vi "TEST SCREEN UPDATE.vi"(0 "Staion  in 1":refnum<k5>, 2 "Staion  in 2":refnum<k5>, 3 "Staion  in error 2":errorcluster, 4 "Staion  in 3":refnum<k5>, 5 "Staion  in error 3":errorcluster, 6 "DataBase connection in":T10, 7 "Database error in":errorcluster, 21 "Staion  in error 1":errorcluster) -> (1 "Staion Error Out 1":errorcluster, 20 "Staion Out 1":refnum<k5>, 22 "Staion Out 2":refnum<k5>, 23 "Staion Error Out 2":errorcluster, 24 "Staion Out 3":refnum<k5>, 25 "Staion Error Out 3":errorcluster, 26 "Database connection out":T10, 27 "Database error out":errorcluster)   [LabVIEW 2024]
uses:
  <vilib>/addons/database/Connection.llb/Conn ObjectReference.ctl
  Controls/OP10_Cluster.ctl
  Controls/OP20_Cluster.ctl
  Controls/OP30_Cluster.ctl
  Controls/OP30_1_Cluster.ctl
  Controls/OP40_1_Cluster.ctl
  Controls/OP40_Cluster.ctl
  Controls/OP40_2_Cluster.ctl
  Controls/OP40_3_Cluster.ctl
  Controls/Data_Cluster_1.ctl
  test sequnece leak.ctl
  test setting.ctl
  Data base/database cluster.ctl
  Variable/Global.vi
  Support/Message Queue/Message Queue.lvlib
  <vilib>/addons/database/NI_Database_API.lvlib
panel:
  in  "Exit":bool
  in  "Tab Control":enum32{"Screen_1", "Screen_2", "Other"}(tab)
  out "OP_30_1":T1
  out "OP_30":T2
  out "OP_20":T3
  out "OP_10":T4
  out "Result":string[][](table)
  out "OP_40_3":T5
  out "OP_40_2":T6
  out "OP_40":T7
  out "OP_40_1":T8
  in  "Tab Control 2":enum32{"OP_10", "OP_20", "OP_30", "OP_40"}(tab)
  out "OP_10":string[](array[string])
  in  "Barcode OK":bool
  in  "Barcode NG":bool
  in  "Barcode Already":bool
  in  "M 1":T9
  out "OP_10":u16[][](array[numeric])
  out "OP_10":sgl[][](array[numeric])
  in  "Barcode Already 2":bool
  in  "Barcode NG 2":bool
  in  "Barcode OK 2":bool
  in  "M 2":T9
  out "OP_20":string[](array[string])
  out "OP_20":u16[][](array[numeric])
  out "OP_20":sgl[][](array[numeric])
  in  "M 3":T9
  in  "Barcode Already 3":bool
  in  "Barcode NG 3":bool
  in  "Barcode OK 3":bool
  out "OP_30":string[](array[string])
  out "OP_30":u16[][](array[numeric])
  out "OP_30":sgl[][](array[numeric])
  in  "M 4":T9
  in  "Barcode Already 4":bool
  in  "Barcode NG 4":bool
  in  "Barcode OK 4":bool
  out "OP_40":string[](array[string])
  out "OP_40":sgl[][](array[numeric])
  out "OP_40":u16[][](array[numeric])
  out "sr. out BARCODE":i32
  out "sr. out Laser":i32
  out "length":i32
  out "CommLoopCount":i32
  out "Communication error 3":bool
  out "Communication error 2":bool
  out "Communication error 1":bool
  out "path for Laser sr":path
  out "path for Barcode sr.":path
  in  "Model NAME":string
  in  "count Path":path=path "D:/Configuration Folder Barcode/srno"
  in  "Visible":bool
  out "Exit 3":bool
  in  "TEST SETTING PATH":path=path "D:/Data Actuator/config/Settings"
  in  "Setting":path=path "D:/data/Test Settings"
  # "Test Screen"
  # "TESTING DATALOGGING SYSTEM"
  # "Station  OP 10"
  # "Station  OP 20"
  # "Station  OP 30"
  # "Station  OP 30_1"
  # "Station  OP 40"
  # "Station  OP 40_1"
  # "Station  OP 40_2"
  # "Station  OP 40_3"
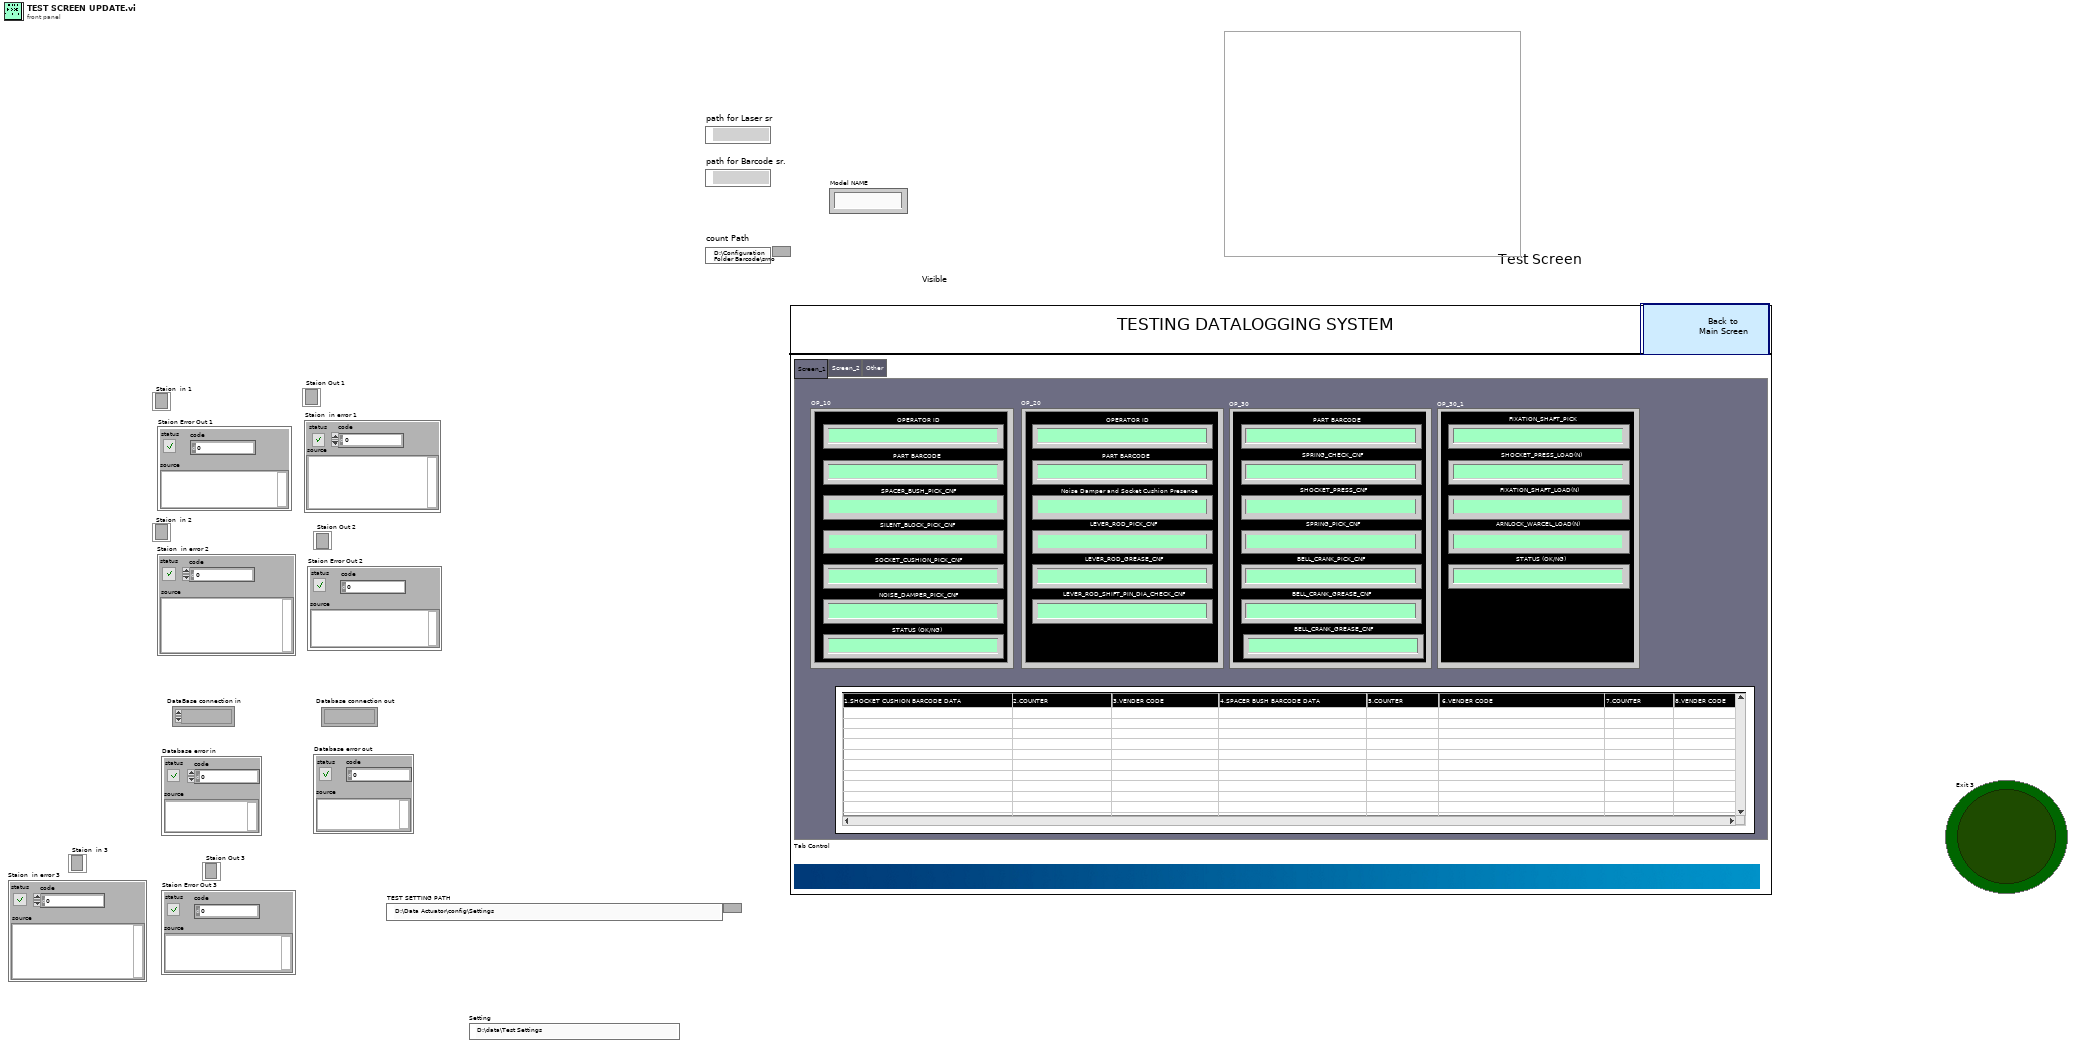
[diagram p1: front panel]
types:
  T1 = typedef "OP30_1_Cluster.ctl" = cluster{"SHOCKET_PRESS_LOAD(N) ":string, "FIXATION_SHAFT_PICK   ":string, "FIXATION_SHAFT_LOAD(N)":string, "ARNLOCK_WARCEL_LOAD(N)":string, "STATUS (OK/NG)":string}
  T2 = typedef "OP30_Cluster.ctl" = cluster{"SPRING_CHECK_CNF ":string, "PART BARCODE  ":string, "SHOCKET_PRESS_CNF":string, "SPRING_PICK_CNF":string, "BELL_CRANK_PICK_CNF":string, "BELL_CRANK_GREASE_CNF":string, "BELL_CRANK_GREASE_CNF":string}
  T3 = typedef "OP20_Cluster.ctl" = cluster{"PART BARCODE ":string, "OPERATOR ID ":string, "Noise Damper and Socket Cushion Presence":string, "LEVER_ROD_PICK_CNF":string, "LEVER_ROD_GREASE_CNF":string, "LEVER_ROD_SHIFT_PIN_DIA_CHECK_CNF":string}
  T4 = typedef "OP10_Cluster.ctl" = cluster{"OPERATOR ID ":string, "PART BARCODE ":string, "SPACER_BUSH_PICK_CNF":string, "SILENT_BLOCK_PICK_CNF":string, "SOCKET_CUSHION_PICK_CNF":string, "NOISE_DAMPER_PICK_CNF":string, "STATUS (OK/NG)":string}
  T5 = typedef "OP40_3_Cluster.ctl" = cluster{"SELECT_5TH_REV_LOAD(N) ":string, "SELECT_1ST_2ND_LOAD(N)":string, "HYSTERISIS CONFIRMATION":string, "PUNCH CONFIRMATION":string, "PDI FIXTURE CONFIRMATION":string, "EOL OK BARCODE SCAN CNF":string, "STATUS (OK/NG)":string}
  T6 = typedef "OP40_2_Cluster.ctl" = cluster{"SHIFT_2ND_4TH_REV_TRAVEL ":string, "PART BARCODE ":string, "SHIFT_1ST_3RD_5TH_TRAVEL ":string, "SHIFT_2ND_4TH_REV_LOAD(N)":string, "SHIFT_1ST_3RD_5TH_LOAD(N)":string, "SELECT_1ST_2ND_TRAVEL":string, "SELECT_5TH_REV_TRAVEL":string}
  T7 = typedef "OP40_Cluster.ctl" = cluster{"PART BARCODE ":string, "OPERATOR ID ":string, "BOOT_ORIENTATION_CHECK_CNF":string, "3_BOND_CONFIRMATION":string, "STATUS (OK/NG)":string, "PRETIGHT ANGLE":string, "POST TIGHT ANGLE":string}
  T8 = typedef "OP40_1_Cluster.ctl" = cluster{"MAX KNOB TORQUE ":string, "KNOB TIGHT BARCODE OK ":string, "NO. OF TURNS":string, "HEIGHT CHECK":string, "2 MM GAUGE CHECK":string, "STATUS (OK/NG)":string, "OPERATOR ID":string}
  T9 = cluster{"Test Start Leak":bool, "Test Stop Leak":bool, "Scan Barcode":bool, "Test Running":bool, "Test OK":bool, "Test NG":bool, "Spare 1":bool, "Spare 2":bool}
  T10 = typedef "NI_Database_API.lvlib/Conn ObjectReference.ctl" = refnum<k1>
  T11 = typedef "Data_Cluster_1.ctl" = cluster{"OP_10":T4}
  T12 = enum16{"open", "replace", "create", "open or create", "replace or create", "replace or create with confirmation"}
  T13 = typedef "test setting.ctl" = cluster{"M&M Part No.":string, "Vendor Code":string, "Part Identification Code":string, "Next Barcode Printing Wait Time":i32, "Path for LAser":path}
  T14 = typedef "test sequnece leak.ctl" = enum16{"Intilize", "CYCLE RESET", "Wait For teststart", "wait for scan", "check Barcode", "wait for start", "Wait for result", "wait for complete", "test stop", "Wait for LAser Scan Data", "check Scan Laser Data", "data save", "update tabel", "send data to Laser", "wait for Laser Start", "wait for laser stop"}
  T15 = typedef "database cluster.ctl" = cluster{"ID":i64, "Datetime":string, "PARTBARCODE":string, "TORQUE":string, "RESULT1":string, "CHILD1":string, "CHILD2":string, "CHILD3":string, "CHILD4":string, "RESULT2":string, "FINALBARCODE":string, "RESULT3":string, "REMARK":string, "OTHER":string}
  T16 = typedef "Communication setting.ctl" = cluster{"Light Scanner Port":refnum<visa-resource-name>, "Shift-A":timestamp, "Shift-B":timestamp, "Shift-C":timestamp, "Leak Scanner Port":refnum<visa-resource-name>, "Barcode Printer":refnum<visa-resource-name>}
  T17 = cluster{"[0]":string, "[1]":string, "[2]":string, "[3]":string, "[4]":string, "[5]":string, "[6]":string}
  T18 = cluster{"M--- 0-7[0]":bool, "M--- 0-7[1]":bool, "M--- 0-7[2]":bool, "M--- 0-7[3]":bool, "M--- 0-7[4]":bool, "M--- 0-7[5]":bool, "M--- 0-7[6]":bool, "M--- 0-7[7]":bool}
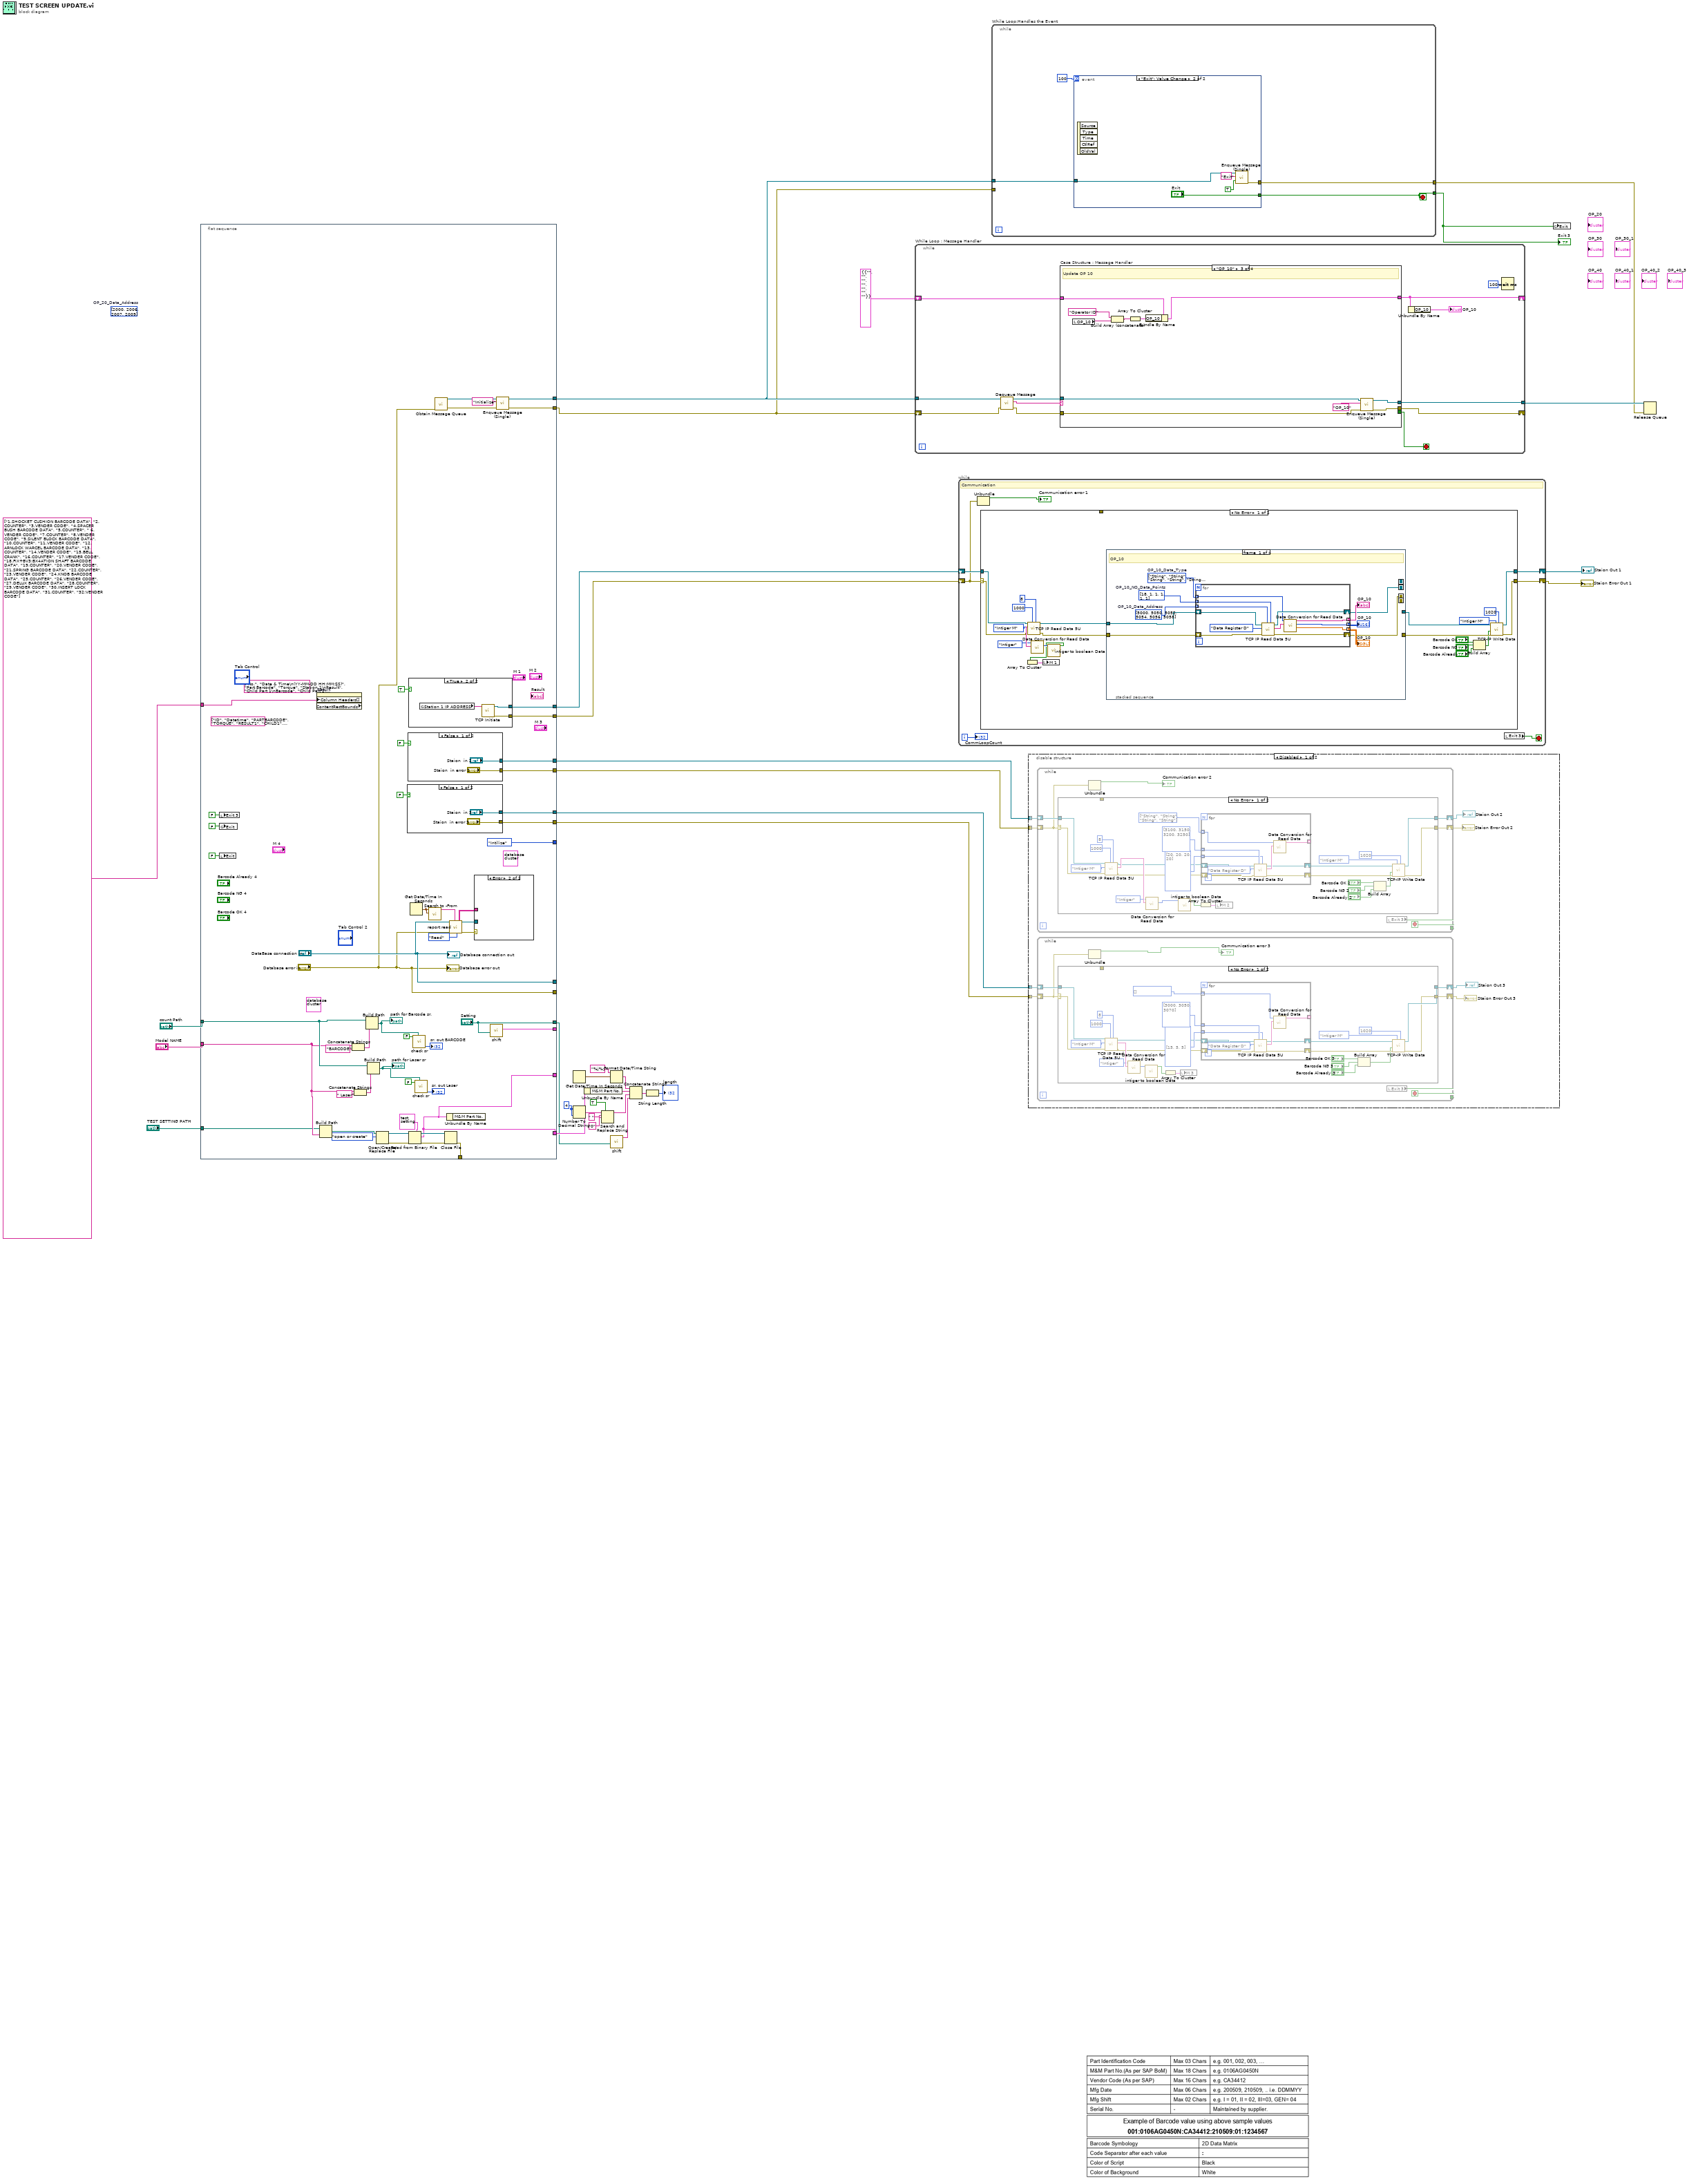
[diagram p0: block diagram]
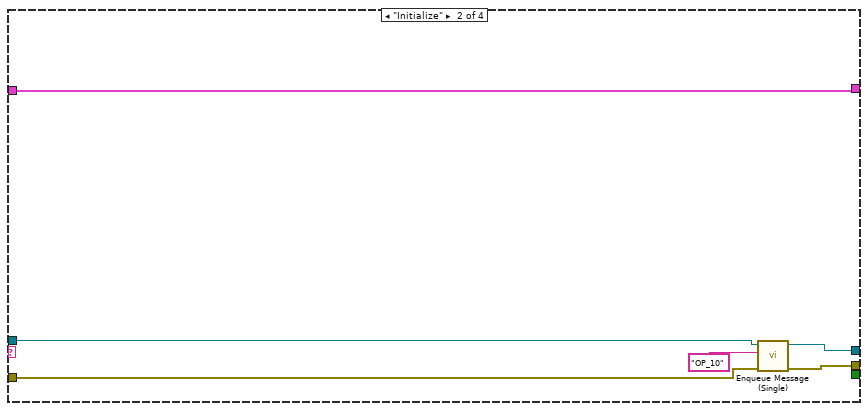
[diagram p3: hidden frame]
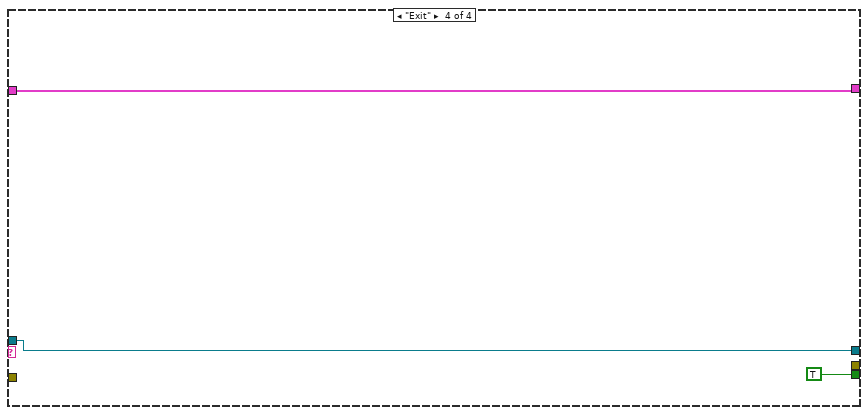
[diagram p4: hidden frame]
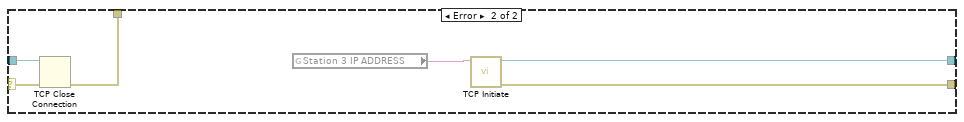
[diagram p5: hidden frame]
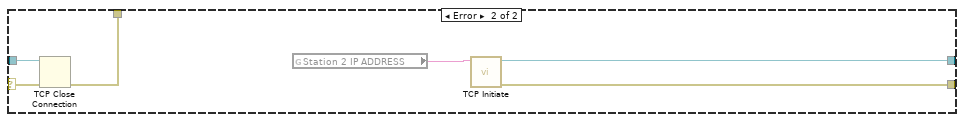
[diagram p6: hidden frame]
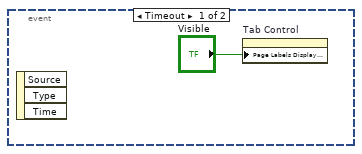
[diagram p8: hidden frame]
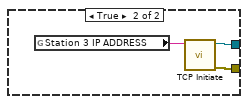
[diagram p9: hidden frame]
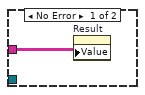
[diagram p10: hidden frame]
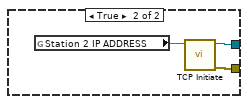
[diagram p11: hidden frame]
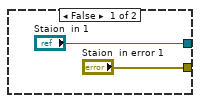
[diagram p12: hidden frame]
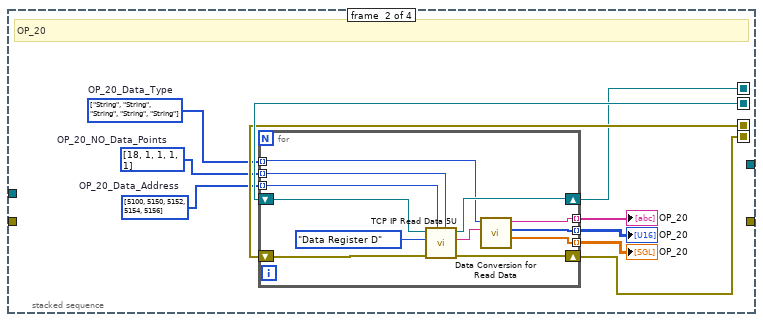
[diagram p13: hidden frame]
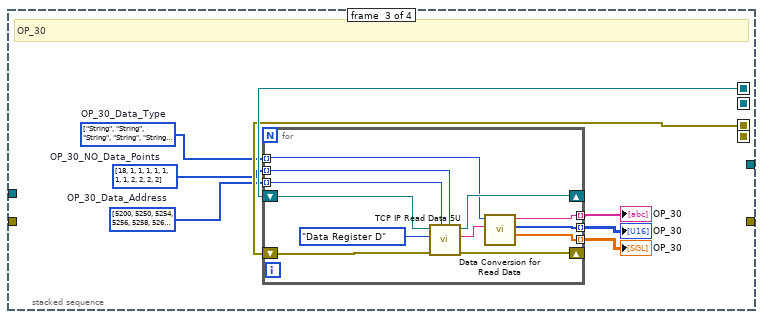
[diagram p14: hidden frame]
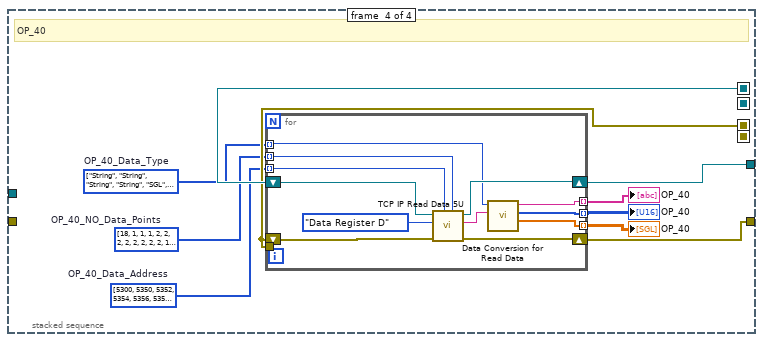
[diagram p15: hidden frame]
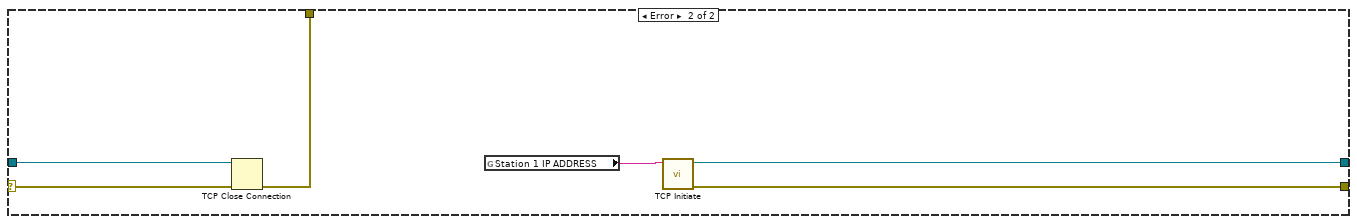
[diagram p16: hidden frame]
diagram:
  (unwired) i32[] [2000, 2006, 2007, 2009]  # OP_20_Data_Address
  w15 = i16 4 ("width (-)")
  n1 = flat-sequence {
    tunnel: ["Setting"] -> w14
    tunnel: [w83] -> _
    tunnel: [w81] -> w31
    tunnel: [w80] -> w30
    tunnel: [test_sequnece_leak."Intilize" ("Enum 2")] -> _
    tunnel: [w74] -> w10
    tunnel: [w73] -> w9
    tunnel: ["DataBase connection in"] -> _
    tunnel: ["Database error in"] -> _
    tunnel: [w60] -> _
    tunnel: [w45] -> _
    tunnel: "count Path" -> [w48]
    tunnel: "Model NAME" -> [w47]
    tunnel: "TEST SETTING PATH" -> [w46]
    tunnel: [w45] -> w16
    tunnel: [w43] -> w8
    tunnel: [w42] -> w7
    tunnel: string[] ["1.SHOCKET CUSHION BARCODE DATA", "2.COUNTER", "3.VENDER CODE", "4.SPACER BUSH BARCODE DATA", "5.COUNTER", " 6.VENDER CODE", "7.COUNTER", "8.VENDER CODE", "9.SILENT BLOCK BARCODE DATA", "10.COUNTER", "11.VENDER CODE", "12.ARNLOCK WARCEL BARCODE DATA", "13.COUNTER", "14.VENDER CODE", "15.BELL CRANK", "16.COUNTER", "17.VENDER CODE", "18.FIX+BV3:BX4ATION SHAFT BARCODE DATA", "19.COUNTER", "20.VENDER CODE", "21.SPRING BARCODE DATA", "22.COUNTER", "23.VENDER CODE", "24.KNOB BARCODE DATA", "25.COUNTER", "26.VENDER CODE", "27.DELUX BARCODE DATA", "28.COUNTER", "29.VENDER CODE", "30.INSERT LOCK BARCODE DATA", "31.COUNTER", "32:VENDER CODE"] ("Column Header Strings[]") -> [w41]
    tunnel: [w37] -> w4
    tunnel: [w35] -> w5
    frame #0 {
      (unwired) string[] ["ID", "Datetime", "PARTBARCODE", "TORQUE", "RESULT1", "CHILD1", "CHILD2", "CHILD3", "CHILD4", "RESULT2", "FINALBARCODE", "RESULT3", "REMARK", "OTHER"] ("tables")
      (unwired) T15 {"ID"=0, "Datetime"="", "PARTBARCODE"="", "TORQUE"="", "RESULT1"="", "CHILD1"="", "CHILD2"="", "CHILD3"="", "CHILD4"="", "RESULT2"="", "FINALBARCODE"="", "RESULT3"="", "REMARK"="", "OTHER"=""} ("Data")
      (unwired) string[] ["No.", "Date & Time\n(YY-MM-DD HH:MM:SS)", "Part Barcode", "Torque", "Station 1\nResult", "Child Part 1\nBarcode", "Child Part 2\nBarcode", "Child Part 3\nBarcode", "Child Part 4\nBarcode", "Station 2\nResult", "Final Part\nBarcode", "Remark", "Other"] ("Column Header Strings[]")
      (unwired) T15 {"ID"=0, "Datetime"="", "PARTBARCODE"="", "TORQUE"="", "RESULT1"="", "CHILD1"="", "CHILD2"="", "CHILD3"="", "CHILD4"="", "RESULT2"="", "FINALBARCODE"="", "RESULT3"="", "REMARK"="", "OTHER"=""} ("Data")
      n2 = local write "Exit 3"(FALSE ("Exit 3")) -> ()
      n3 = global write "Global.vi" "Exit"(FALSE ("Exit")) -> ()
      n4 = local write "Exit"(FALSE ("Exit")) -> ()
      n5 = property on="Result" class="Tbl (strict)" props=["Column Headers[]", "ContentRectBounds"]("Column Headers[]"=w41) -> ()  [unwired: 2 in, 3 out]
      n6 = Build Path(base path=w46, name or relative path=w47) -> (appended path=w62:path)
      n7 = Concatenate Strings(w47, "BARCODE" ("string")) -> (w68:string)
      n8 = Concatenate Strings(w47, " Laser" ("string")) -> (w53:string)
      n9 = Build Path(base path=w48, name or relative path=w68) -> (appended path=w69:path)
      "path for Barcode sr." <- w69
      n10 = Build Path(base path=w48, name or relative path=w53) -> (appended path=w52:path)
      "path for Laser sr" <- w52
      n11 = Open/Create/Replace File(file path (use dialog)=w62, operation (0:open)=T12."open or create") -> (refnum out=w67:refnum<file>, error out=w66:errorcluster)  [unwired: 4 in, 1 out]
      n12 = case shown="False" FALSE {
        tunnel: ["Staion  in 3" w89] -> w43
        tunnel: ["Staion  in error 3" w88] -> w42
        frame False {
        }
        frame True {
          n13 = global read "Global.vi" "Station 3 IP ADDRESS"() -> (w87:string)
          n14 = call "TCP Initiate.vi"("IP ADDRESS"=w87) -> ("error out"=w88:errorcluster, "connection ID"=w89:refnum<k5>)  [unwired: 9 in]
        }
      }
      n15 = case shown="False" FALSE {
        tunnel: ["Staion  in 2" w95] -> w74
        tunnel: ["Staion  in error 2" w94] -> w73
        frame False {
        }
        frame True {
          n16 = global read "Global.vi" "Station 2 IP ADDRESS"() -> (w93:string)
          n17 = call "TCP Initiate.vi"("IP ADDRESS"=w93) -> ("error out"=w94:errorcluster, "connection ID"=w95:refnum<k5>)  [unwired: 9 in]
        }
      }
      n18 = Read from Binary File(5:T13 {"M&M Part No."="", "Vendor Code"="02BHMSI1009190338RKWPG", "Part Identification Code"="02CRMTT1009190250KWPG", "Next Barcode Printing Wait Time"=0, "Path for LAser"=path ""} ("Cluster"), 8:w66, 11:w67) -> (0:w65:errorcluster, 2:w45:T13, 3:w64:refnum<file>)  [unwired: 3 in, 1 out]
      n19 = case shown="True" TRUE {
        tunnel: ["Staion  in 1" w100] -> w81
        tunnel: ["Staion  in error 1" w99] -> w80
        frame False {
        }
        frame True {
          n20 = global read "Global.vi" "Station 1 IP ADDRESS"() -> (w98:string)
          n21 = call "TCP Initiate.vi"("IP ADDRESS"=w98) -> ("error out"=w99:errorcluster, "connection ID"=w100:refnum<k5>)  [unwired: 9 in]
        }
      }
      n22 = Get Date/Time In Seconds() -> (seconds since 1Jan1904=w59:timestamp)
      n23 = call "check sr.vi"("file path (use dialog)"=w69, "writeL:t"=FALSE) -> ("sr. out"=→"sr. out BARCODE":i32)  [unwired: 9 in]
      n24 = call "check sr.vi"("file path (use dialog)"=w52, "writeL:t"=FALSE) -> ("sr. out"=→"sr. out Laser":i32)  [unwired: 9 in]
      n25 = call "Search to -From.vi"("From date"=w59, "To Date"=w59) -> ("search dataString"=w57:string)  [unwired: 9 in]
      n26 = call "Obtain Message Queue.vi"("error in (no error)"="Database error in") -> ("error out"=w38:errorcluster, "Message Queue"=w36:refnum<queue>)  [unwired: 9 in]
      n27 = Close File(refnum=w64, error in=w65) -> (error out=w60:errorcluster)  [unwired: 1 out]
      n28 = Unbundle By Name(w45) -> ()  [unwired: 1 out]
      n29 = call "report read.vi"("connection reference"="DataBase connection in", "error in (no error)"="Database error in", "search dataString"=w57, "Enum"=enum16{"Write", "Read"}."Read") -> ("Search Reverse"=w56:string[][], "connection reference out"=w55:T10, "error out"=w40:errorcluster)  [unwired: 10 in, 3 out]
      n30 = case shown="Error" w40 {
        tunnel: w56 -> [w90 _]
        tunnel: w55 -> [_ _]
        frame No Error {
          n31 = property on="Result" class="Tbl (strict)"("Value"=w90) -> ()  [unwired: 2 in, 2 out]
        }
        frame Error {
        }
      }
      n32 = call "shift.vi"("Setting"="Setting") -> ("data"=w83:T16)  [unwired: 9 in, 1 out]
      n33 = call "Enqueue Message (Single).vi"("error in (no error)"=w38, "Message"="Initialize", "Message Queue"=w36) -> ("error out"=w37:errorcluster, "dup Message Queue"=w35:refnum<queue>)  [unwired: 7 in]
      "Database connection out" <- "DataBase connection in"
      "Database error out" <- "Database error in"
    }
  }
  n34 = Get Date/Time In Seconds() -> (seconds since 1Jan1904=w21:timestamp)
  n35 = Number To Decimal String(number=w15, width (-)=w15) -> (decimal integer string=w17:string)
  n36 = Unbundle By Name(w16) -> ("M&M Part No."=w25:string)
  n37 = Search and Replace String(replace all?=TRUE ("replace all? (F)"), input string=w17, search string=" ", replace string="0" ("replace string (\"\")")) -> (result string=w20:string)  [unwired: 4 in, 3 out]
  n38 = Format Date/Time String(time format string (%c)="%j%y", seconds (now)=w21) -> (date/time string=w24:string)  [unwired: 1 in]
  n39 = call "shift.vi"("Setting"=w14) -> ("SHIFT_A"=w13:string)  [unwired: 9 in, 1 out]
  n40 = Concatenate Strings(w24, w25, w20, w13) -> (w12:string)
  n41 = String Length(string=w12) -> (length=→"length":i32)
  n42 = while "While Loop : Message Handler" {
    tunnel: w5 -> [w111]
    tunnel: [w106] -> w3
    shift-right: [w104] -> _
    shift-left: w4 -> [w112]
    shift-right: [w102] -> _
    shift-left: T11 {"OP_10"={"OPERATOR ID "="", "PART BARCODE "="", "SPACER_BUSH_PICK_CNF"="", "SILENT_BLOCK_PICK_CNF"="", "SOCKET_CUSHION_PICK_CNF"="", "NOISE_DAMPER_PICK_CNF"="", "STATUS (OK/NG)"=""}} ("Data Cluster") -> [w103]
    stop <- w107 stop-if-true
    n43 = call "Dequeue Message.vi"("error in (no error)"=w112, "Message Queue"=w111) -> ("error out"=w110:errorcluster, "Message"=w109:string, "dup Message Queue"=w108:refnum<queue>)  [unwired: 6 in, 1 out]
    n44 = case "Case Structure : Message Handler" shown="\"OP_10\"" w109 {
      tunnel: w110 -> [_ w120 w131 _]
      tunnel: w108 -> [w114 w117 w128 w133]
      tunnel: [_ _ _ TRUE] -> w107
      tunnel: [w114 w116 w127 w133] -> w106
      tunnel: [_ w119 w130 _] -> w104
      tunnel: w103 -> [w113 w115 w122 w132]
      tunnel: [w113 w115 w121 w132] -> w102
      frame "False", Default {
      }
      frame "Initialize" {
        n45 = call "Enqueue Message (Single).vi"("error in (no error)"=w120, "Message"="OP_10", "Message Queue"=w117) -> ("error out"=w119:errorcluster, "dup Message Queue"=w116:refnum<queue>)  [unwired: 7 in]
      }
      frame "OP_10" {
        # "Update OP 10"
        n46 = local read "OP_10"() -> (w126:string[])
        n47 = Build Array (concatenate)("Operator ID", w126) -> (w124:string[])
        n48 = Array To Cluster(array=w124) -> (cluster=w123:T17)
        n49 = Bundle By Name(cluster=w122, "OP_10"=w123) -> (w121:T11)
        n50 = call "Enqueue Message (Single).vi"("error in (no error)"=w131, "Message"="OP_10", "Message Queue"=w128) -> ("error out"=w130:errorcluster, "dup Message Queue"=w127:refnum<queue>)  [unwired: 7 in]
      }
      frame "Exit" {
      }
    }
    n51 = Unbundle By Name(w102) -> ("OP_10"=→"OP_10":T4)
    n52 = Wait (ms)(milliseconds to wait=u32 100) -> ()  [unwired: 1 out]
  }
  n53 = while {
    shift-right: [w141] -> w33
    shift-left: w31 -> [w140]
    shift-right: [w139] -> w32
    shift-left: w30 -> [w138]
    i -> [w135]
    stop <- w137 stop-if-true
    # "Communication"
    n54 = Unbundle(w138) -> ("status"=→"Communication error 1":bool)  [unwired: 2 out]
    n55 = case shown="No Error" w138 {
      selector: w138 -> [w156 w253]
      tunnel: [w146 w255] -> w141
      tunnel: [w145 w254] -> w139
      tunnel: w140 -> [w157 w252]
      tunnel: [_ w251] -> _
      frame No Error {
        n56 = call "TCP IP Read Data 5U.vi"("No of data regiter read"=8, "Start Address"=1000, "error in"=w156, "Data Rigister/Memory"=enum16{"Data Register D", "Intiger M"}."Intiger M", "connection ID"=w157) -> ("error out"=w147:errorcluster, "RAw Data"=w162:string, "connection ID Out"=w148:refnum<k5>)  [unwired: 4 in]
        n57 = call "Data Conversion for Read Data.vi"("data out"=w162, "Read Data Type"=enum16{"String", "Intiger", "DBL"}."Intiger") -> ("M Intiger"=w163:u16[])  [unwired: 6 in, 3 out]
        n58 = call "intiger to boolean Data.vi"("data"=w163) -> ("M--- 0-7"=w143:bool[])  [unwired: 9 in, 5 out]
        n59 = Array To Cluster(array=w143) -> (cluster=w142:T18)
        n60 = local write "M 1"(w142) -> ()
        n61 = stacked-sequence {
          seq-local: [w168 _ _ _] -> [_ w195 _ _]
          seq-local: [w167 _ _ _] -> [_ w194 w214 w234]
          seq-local: [_ w187 _ _] -> [_ _ w215 w237]
          seq-local: [_ w186 _ _] -> [_ _ _ _]
          tunnel: [_ _ _ w236] -> w155
          tunnel: [_ _ _ w235] -> w154
          tunnel: w148 -> [w173 _ _ _]
          tunnel: w147 -> [w172 _ _ _]
          frame #0 {
            w164 = i32[] [5000, 5050, 5052, 5054, 5056, 5058]  # OP_10_Data_Address
            w165 = i32[] [18, 1, 1, 1, 1, 1]  # OP_10_NO_Data_Points
            w166 = enum16{"String", "Intiger", "DBL", "SGL"}[] [enum."String", enum."String", enum."String", enum."String", enum."String", enum."String"] items=["String", "Intiger", "DBL", "SGL"]  # OP_10_Data_Type
            # "OP_10"
            n62 = for {
              tunnel: [w179] -> w169 mode=indexing
              shift-right: [w181] -> w168
              shift-left: w173 -> [w183]
              shift-right: [w180] -> w167
              shift-left: w172 -> [w182]
              tunnel: w164 -> [w178] mode=indexing
              tunnel: w165 -> [w177] mode=indexing
              tunnel: [w176] -> w170 mode=indexing
              tunnel: [w175] -> w171 mode=indexing
              tunnel: w166 -> [w174] mode=indexing
              n63 = call "TCP IP Read Data 5U.vi"("No of data regiter read"=w177, "Start Address"=w178, "error in"=w182, "Data Rigister/Memory"=enum16{"Data Register D", "Intiger M"}."Data Register D", "connection ID"=w183) -> ("error out"=w180:errorcluster, "RAw Data"=w184:string, "connection ID Out"=w181:refnum<k5>)  [unwired: 4 in]
              n64 = call "Data Conversion for Read Data.vi"("data out"=w184, "Read Data Type"=w174) -> ("Data regiter"=w176:sgl[], "M Intiger"=w175:u16[], "String"=w179:string)  [unwired: 6 in, 1 out]
            }
            "OP_10" <- w169
            "OP_10" <- w171
            "OP_10" <- w170
          }
          frame #1 {
            w191 = enum16{"String", "Intiger", "DBL", "SGL"}[] [enum."String", enum."String", enum."String", enum."String", enum."String"] items=["String", "Intiger", "DBL", "SGL"]  # OP_20_Data_Type
            w192 = i32[] [18, 1, 1, 1, 1]  # OP_20_NO_Data_Points
            w193 = i32[] [5100, 5150, 5152, 5154, 5156]  # OP_20_Data_Address
            # "OP_20"
            n65 = for {
              tunnel: [w201] -> w190 mode=indexing
              shift-right: [w203] -> w187
              shift-left: w195 -> [w205]
              shift-right: [w202] -> w186
              shift-left: w194 -> [w204]
              tunnel: w193 -> [w200] mode=indexing
              tunnel: w192 -> [w199] mode=indexing
              tunnel: [w198] -> w188 mode=indexing
              tunnel: [w197] -> w189 mode=indexing
              tunnel: w191 -> [w196] mode=indexing
              n66 = call "TCP IP Read Data 5U.vi"("No of data regiter read"=w199, "Start Address"=w200, "error in"=w204, "Data Rigister/Memory"=enum16{"Data Register D", "Intiger M"}."Data Register D", "connection ID"=w205) -> ("error out"=w202:errorcluster, "RAw Data"=w206:string, "connection ID Out"=w203:refnum<k5>)  [unwired: 4 in]
              n67 = call "Data Conversion for Read Data.vi"("data out"=w206, "Read Data Type"=w196) -> ("Data regiter"=w198:sgl[], "M Intiger"=w197:u16[], "String"=w201:string)  [unwired: 6 in, 1 out]
            }
            "OP_20" <- w190
            "OP_20" <- w189
            "OP_20" <- w188
          }
          frame #2 {
            w208 = enum16{"String", "Intiger", "DBL", "SGL"}[] [enum."String", enum."String", enum."String", enum."String", enum."String", enum."String", enum."String", enum."String", enum."SGL", enum."SGL", enum."SGL", enum."String"] items=["String", "Intiger", "DBL", "SGL"]  # OP_30_Data_Type
            w209 = i32[] [18, 1, 1, 1, 1, 1, 1, 1, 2, 2, 2, 2]  # OP_30_NO_Data_Points
            w210 = i32[] [5200, 5250, 5254, 5256, 5258, 5260, 5262, 5264, 5266, 5268, 5270, 5272]  # OP_30_Data_Address
            # "OP_30"
            n68 = for {
              tunnel: [w221] -> w213 mode=indexing
              shift-right: [w223] -> _
              shift-left: w215 -> [w225]
              shift-right: [w222] -> _
              shift-left: w214 -> [w224]
              tunnel: w210 -> [w220] mode=indexing
              tunnel: w209 -> [w219] mode=indexing
              tunnel: [w218] -> w211 mode=indexing
              tunnel: [w217] -> w212 mode=indexing
              tunnel: w208 -> [w216] mode=indexing
              n69 = call "TCP IP Read Data 5U.vi"("No of data regiter read"=w219, "Start Address"=w220, "error in"=w224, "Data Rigister/Memory"=enum16{"Data Register D", "Intiger M"}."Data Register D", "connection ID"=w225) -> ("error out"=w222:errorcluster, "RAw Data"=w226:string, "connection ID Out"=w223:refnum<k5>)  [unwired: 4 in]
              n70 = call "Data Conversion for Read Data.vi"("data out"=w226, "Read Data Type"=w216) -> ("Data regiter"=w218:sgl[], "M Intiger"=w217:u16[], "String"=w221:string)  [unwired: 6 in, 1 out]
            }
            "OP_30" <- w213
            "OP_30" <- w212
            "OP_30" <- w211
          }
          frame #3 {
            w231 = enum16{"String", "Intiger", "DBL", "SGL"}[] [enum."String", enum."String", enum."String", enum."String", enum."SGL", enum."SGL", enum."String", enum."SGL", enum."SGL", enum."String", enum."String", enum."String", enum."String", enum."SGL", enum."SGL", enum."Intiger", enum."Intiger", enum."SGL", enum."SGL", enum."SGL", enum."SGL", enum."SGL", enum."String", enum."String", enum."String", enum."String", enum."String"] items=["String", "Intiger", "DBL", "SGL"]  # OP_40_Data_Type
            w232 = i32[] [18, 1, 1, 1, 2, 2, 2, 2, 2, 2, 2, 2, 18, 2, 2, 2, 2, 2, 2, 2, 2, 2, 1, 1, 1, 1, 18]  # OP_40_NO_Data_Points
            w233 = i32[] [5300, 5350, 5352, 5354, 5356, 5358, 5360, 5362, 5364, 5366, 5368, 5370, 5400, 5450, 5452, 5456, 5458, 5460, 5462, 5464, 5466, 5468, 6570, 5472, 5474, 5476, 5500]  # OP_40_Data_Address
            # "OP_40"
            n71 = for {
              tunnel: [w243] -> w230 mode=indexing
              shift-right: [w245] -> w236
              shift-left: w237 -> [w247]
              shift-right: [w244] -> w235
              shift-left: w234 -> [w246]
              tunnel: w233 -> [w242] mode=indexing
              tunnel: w232 -> [w241] mode=indexing
              tunnel: [w240] -> w228 mode=indexing
              tunnel: [w239] -> w229 mode=indexing
              tunnel: w231 -> [w238] mode=indexing
              tunnel: w234 -> [_]
              n72 = call "TCP IP Read Data 5U.vi"("No of data regiter read"=w241, "Start Address"=w242, "error in"=w246, "Data Rigister/Memory"=enum16{"Data Register D", "Intiger M"}."Data Register D", "connection ID"=w247) -> ("error out"=w244:errorcluster, "RAw Data"=w248:string, "connection ID Out"=w245:refnum<k5>)  [unwired: 4 in]
              n73 = call "Data Conversion for Read Data.vi"("data out"=w248, "Read Data Type"=w238) -> ("Data regiter"=w240:sgl[], "M Intiger"=w239:u16[], "String"=w243:string)  [unwired: 6 in, 1 out]
            }
            "OP_40" <- w230
            "OP_40" <- w229
            "OP_40" <- w228
          }
        }
        n74 = Build Array("Barcode OK", "Barcode NG", "Barcode Already") -> (w152:bool[])
        n75 = call "TCP-IP Write Data.vi"("Start address"=1020, "Data Rigister/Memory"=enum16{"Data Register D", "Intiger M"}."Intiger M", "error in (no error)"=w154, "M 16 bit Only"=w152, "connection ID"=w155) -> ("error out"=w145:errorcluster, "connection ID out"=w146:refnum<k5>)  [unwired: 5 in]
      }
      frame Error {
        n76 = TCP Close Connection(connection ID=w252, error in (no error)=w253) -> (error out=w251:errorcluster)  [unwired: 1 in, 1 out]
        n77 = global read "Global.vi" "Station 1 IP ADDRESS"() -> (w250:string)
        n78 = call "TCP Initiate.vi"("IP ADDRESS"=w250) -> ("error out"=w254:errorcluster, "connection ID"=w255:refnum<k5>)  [unwired: 9 in]
      }
    }
    n79 = local read "Exit 3"() -> (w137:bool)
    "CommLoopCount" <- w135
  }
  "Staion Out 1" <- w33
  "Staion Error Out 1" <- w32
  n80 = while "While Loop:Handles the Event" {
    tunnel: [w258] -> w29
    tunnel: w5 -> [w257]
    tunnel: w4 -> [_]
    tunnel: [w256] -> w2
    stop <- w258 stop-if-true
    n81 = event shown="[1] \"Exit\": Value Change" {
      selector: _ -> [_ _]
      dyn-events: _ -> [_ _]
      timeout: 100 -> [_ _]
      tunnel: [_ "Exit"] -> w258
      tunnel: w257 -> [_ w263]
      tunnel: [_ w261] -> w256
      event Timeout {
        n82 = event-data() -> ()  [unwired: 1 in, 3 out]
        n83 = property on="Tab Control" class="TabCtl (strict)"("Page Labels Display Visible?"="Visible") -> ()  [unwired: 2 in, 2 out]
      }
      event "Exit": Value Change {
        n84 = event-data() -> ()  [unwired: 1 in, 5 out]
        n85 = call "Enqueue Message (Single).vi"("Priority Message? (F)"=TRUE, "Message"="Exit", "Message Queue"=w263) -> ("error out"=w261:errorcluster)  [unwired: 7 in, 1 out]
      }
    }
  }
  "Exit 3" <- w29
  n86 = disable-structure shown="Disabled" {
    disable-tunnel: w10 -> [w271 _]
    disable-tunnel: w9 -> [w270 _]
    disable-tunnel: w8 -> [w269 _]
    disable-tunnel: w7 -> [w268 _]
    frame Disabled {
      n87 = while {
        tunnel: [w323] -> _
        shift-right: [w327] -> w273
        shift-left: w271 -> [w326]
        shift-right: [w325] -> w272
        shift-left: w270 -> [w324]
        stop <- w323 stop-if-true
        n88 = case shown="No Error" w324 {
          selector: w324 -> [w346 w367]
          tunnel: [w334 w369] -> w327
          tunnel: [w333 w368] -> w325
          tunnel: w326 -> [w347 w366]
          tunnel: [_ w365] -> _
          frame No Error {
            w329 = enum16{"String", "Intiger", "DBL", "SGL"}[] [enum."String", enum."String", enum."String", enum."String"] items=["String", "Intiger", "DBL", "SGL"]
            n89 = call "TCP IP Read Data 5U.vi"("No of data regiter read"=8, "Start Address"=1000, "error in"=w346, "Data Rigister/Memory"=enum16{"Data Register D", "Intiger M"}."Intiger M", "connection ID"=w347) -> ("error out"=w335:errorcluster, "RAw Data"=w352:string, "connection ID Out"=w336:refnum<k5>)  [unwired: 4 in]
            n90 = call "Data Conversion for Read Data.vi"("data out"=w352, "Read Data Type"=enum16{"String", "Intiger", "DBL"}."Intiger") -> ("M Intiger"=w353:u16[])  [unwired: 6 in, 3 out]
            n91 = call "intiger to boolean Data.vi"("data"=w353) -> ("M--- 0-7"=w331:bool[])  [unwired: 9 in, 5 out]
            n92 = Array To Cluster(array=w331) -> (cluster=w330:T18)
            n93 = for {
              tunnel: [w357] -> w328 mode=indexing
              shift-right: [w359] -> w345
              shift-left: w336 -> [w361]
              shift-right: [w358] -> w344
              shift-left: w335 -> [w360]
              tunnel: i32[] [3100, 3150, 3200, 3250] -> [w356] mode=indexing
              tunnel: i32[] [20, 20, 20, 20] ("No of data regiter read") -> [w355] mode=indexing
              tunnel: w329 -> [w354] mode=indexing
              n94 = call "TCP IP Read Data 5U.vi"("No of data regiter read"=w355, "Start Address"=w356, "error in"=w360, "Data Rigister/Memory"=enum16{"Data Register D", "Intiger M"}."Data Register D", "connection ID"=w361) -> ("error out"=w358:errorcluster, "RAw Data"=w362:string, "connection ID Out"=w359:refnum<k5>)  [unwired: 4 in]
              n95 = call "Data Conversion for Read Data.vi"("data out"=w362, "Read Data Type"=w354) -> ("String"=w357:string)  [unwired: 6 in, 3 out]
            }
            n96 = local write "M 2"(w330) -> ()
            n97 = Build Array("Barcode OK 2", "Barcode NG 2", "Barcode Already 2") -> (w342:bool[])
            n98 = call "TCP-IP Write Data.vi"("Start address"=1020, "Data Rigister/Memory"=enum16{"Data Register D", "Intiger M"}."Intiger M", "error in (no error)"=w344, "M 16 bit Only"=w342, "connection ID"=w345) -> ("error out"=w333:errorcluster, "connection ID out"=w334:refnum<k5>)  [unwired: 5 in]
          }
          frame Error {
            n99 = TCP Close Connection(connection ID=w366, error in (no error)=w367) -> (error out=w365:errorcluster)  [unwired: 1 in, 1 out]
            n100 = global read "Global.vi" "Station 2 IP ADDRESS"() -> (w364:string)
            n101 = call "TCP Initiate.vi"("IP ADDRESS"=w364) -> ("error out"=w368:errorcluster, "connection ID"=w369:refnum<k5>)  [unwired: 9 in]
          }
        }
        n102 = Unbundle(w324) -> ("status"=→"Communication error 2":bool)  [unwired: 2 out]
        n103 = local read "Exit 3"() -> (w323:bool)
      }
      "Staion Out 2" <- w273
      "Staion Error Out 2" <- w272
      n104 = while {
        tunnel: [w275] -> _
        shift-right: [w279] -> w267
        shift-left: w269 -> [w278]
        shift-right: [w277] -> w266
        shift-left: w268 -> [w276]
        stop <- w275 stop-if-true
        n105 = case shown="No Error" w276 {
          selector: w276 -> [w298 w319]
          tunnel: [w286 w321] -> w279
          tunnel: [w285 w320] -> w277
          tunnel: w278 -> [w299 w318]
          tunnel: [_ w317] -> _
          frame No Error {
            w280 = enum16{"String", "Intiger", "DBL", "SGL"}[] [] items=["String", "Intiger", "DBL", "SGL"]
            n106 = call "TCP IP Read Data 5U.vi"("No of data regiter read"=8, "Start Address"=1000, "error in"=w298, "Data Rigister/Memory"=enum16{"Data Register D", "Intiger M"}."Intiger M", "connection ID"=w299) -> ("error out"=w287:errorcluster, "RAw Data"=w304:string, "connection ID Out"=w288:refnum<k5>)  [unwired: 4 in]
            n107 = call "Data Conversion for Read Data.vi"("data out"=w304, "Read Data Type"=enum16{"String", "Intiger", "DBL"}."Intiger") -> ("M Intiger"=w305:u16[])  [unwired: 6 in, 3 out]
            n108 = call "intiger to boolean Data.vi"("data"=w305) -> ("M--- 0-7"=w283:bool[])  [unwired: 9 in, 5 out]
            n109 = Array To Cluster(array=w283) -> (cluster=w282:T18)
            n110 = local write "M 3"(w282) -> ()
            n111 = for {
              tunnel: [w309] -> w281 mode=indexing
              shift-right: [w311] -> w297
              shift-left: w288 -> [w313]
              shift-right: [w310] -> w296
              shift-left: w287 -> [w312]
              tunnel: i32[] [3000, 3050, 3070] -> [w308] mode=indexing
              tunnel: i32[] [15, 5, 5] ("No of data regiter read") -> [w307] mode=indexing
              tunnel: w280 -> [w306] mode=indexing
              n112 = call "TCP IP Read Data 5U.vi"("No of data regiter read"=w307, "Start Address"=w308, "error in"=w312, "Data Rigister/Memory"=enum16{"Data Register D", "Intiger M"}."Data Register D", "connection ID"=w313) -> ("error out"=w310:errorcluster, "RAw Data"=w314:string, "connection ID Out"=w311:refnum<k5>)  [unwired: 4 in]
              n113 = call "Data Conversion for Read Data.vi"("data out"=w314, "Read Data Type"=w306) -> ("String"=w309:string)  [unwired: 6 in, 3 out]
            }
            n114 = Build Array("Barcode OK 3", "Barcode NG 3", "Barcode Already 3") -> (w294:bool[])
            n115 = call "TCP-IP Write Data.vi"("Start address"=1020, "Data Rigister/Memory"=enum16{"Data Register D", "Intiger M"}."Intiger M", "error in (no error)"=w296, "M 16 bit Only"=w294, "connection ID"=w297) -> ("error out"=w285:errorcluster, "connection ID out"=w286:refnum<k5>)  [unwired: 5 in]
          }
          frame Error {
            n116 = TCP Close Connection(connection ID=w318, error in (no error)=w319) -> (error out=w317:errorcluster)  [unwired: 1 in, 1 out]
            n117 = global read "Global.vi" "Station 3 IP ADDRESS"() -> (w316:string)
            n118 = call "TCP Initiate.vi"("IP ADDRESS"=w316) -> ("error out"=w320:errorcluster, "connection ID"=w321:refnum<k5>)  [unwired: 9 in]
          }
        }
        n119 = Unbundle(w276) -> ("status"=→"Communication error 3":bool)  [unwired: 2 out]
        n120 = local read "Exit 3"() -> (w275:bool)
      }
      "Staion Out 3" <- w267
      "Staion Error Out 3" <- w266
    }
    frame Enabled {
    }
  }
  n121 = global write "Global.vi" "Exit"(w29) -> ()
  n122 = Release Queue(queue=w3, error in (no error)=w2) -> ()  [unwired: 1 in, 3 out]
